vi "Read Simulated.vi"(8 "error in (no error)":errorcluster, 11 "Init Parameters in":refnum<class "%DEVICE% Init Parameters.lvclass">) -> (0 "error out":errorcluster, 2 "Simulated":bool, 3 "Init Parameters out":refnum<class "%DEVICE% Init Parameters.lvclass">)   [LabVIEW 2017, in "%DEVICE% Messaging.lvlib" / "%DEVICE% Init Parameters.lvclass"]
uses:
  %DEVICE% Init Parameters.lvclass
  %DEVICE% Init Parameters.lvclass/%DEVICE% Init Parameters.ctl
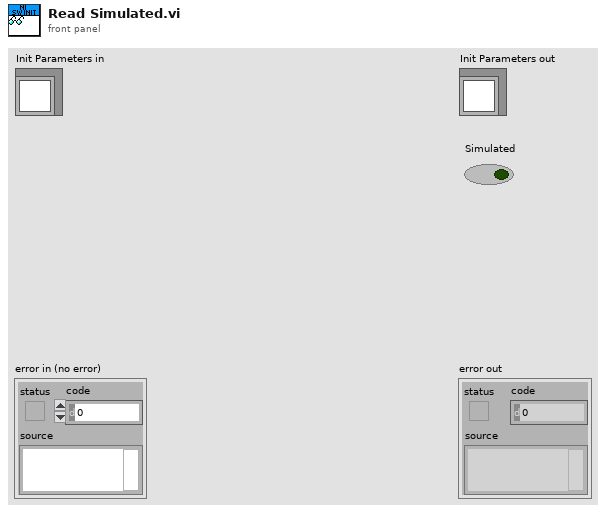
[diagram p1: front panel]
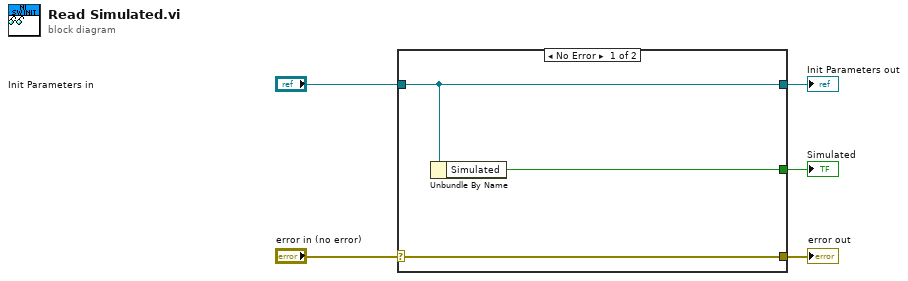
[diagram p0: block diagram]
diagram:
  n1 = case shown="No Error" "error in (no error)" {
    selector: "error in (no error)" -> [w8 w9]
    tunnel: [w8 w9] -> w4
    tunnel: [w7 w10] -> w2
    tunnel: "Init Parameters in" -> [w7 w10]
    tunnel: [w6 _] -> w1
    frame No Error {
      n2 = Unbundle By Name(w7) -> ("Simulated"=w6:bool)
    }
    frame Error {
    }
  }
  "error out" <- w4
  "Init Parameters out" <- w2
  "Simulated" <- w1
